vi "Auto_Routine_RightTwoPieceTRAJ.vi"   [LabVIEW 2023]
uses:
  Shoulder/ShoulderGetSetpointEnum.ctl
  Trajectory/TrajectoryGlobals.vi
  <vilib>/Rock Robotics/WPI/ThirdParty/JAS_Junk/TrajLib/Trajectory_Library.lvlib
types:
  T1 = typedef "ShoulderGetSetpointEnum.ctl" = enum16{"ShoulderRest", "ShoulderSpeaker", "ShoulderAmp"}
  T2 = typedef "Trajectory_Library.lvlib/TRAJECTORY.ctl" = cluster{"TotalTImeSecs":dbl, "States":T3[]}
  T3 = typedef "Trajectory_Library.lvlib/TRAJ_STATE.ctl" = cluster{"TimeSeconds":dbl, "Velocity":dbl, "Acceleration":dbl, "POSE":T4, "Curvature":dbl}
  T4 = typedef "Trajectory_Library.lvlib/POSE2D.ctl" = cluster{"TRANSLATION":T5, "ROTATION":T6}
  T5 = typedef "Trajectory_Library.lvlib/TRANSLATION2D.ctl" = cluster{"X":dbl, "Y":dbl}
  T6 = typedef "Trajectory_Library.lvlib/ROTATION2D.ctl" = cluster{"VALUE":dbl, "COS":dbl, "SIN":dbl}
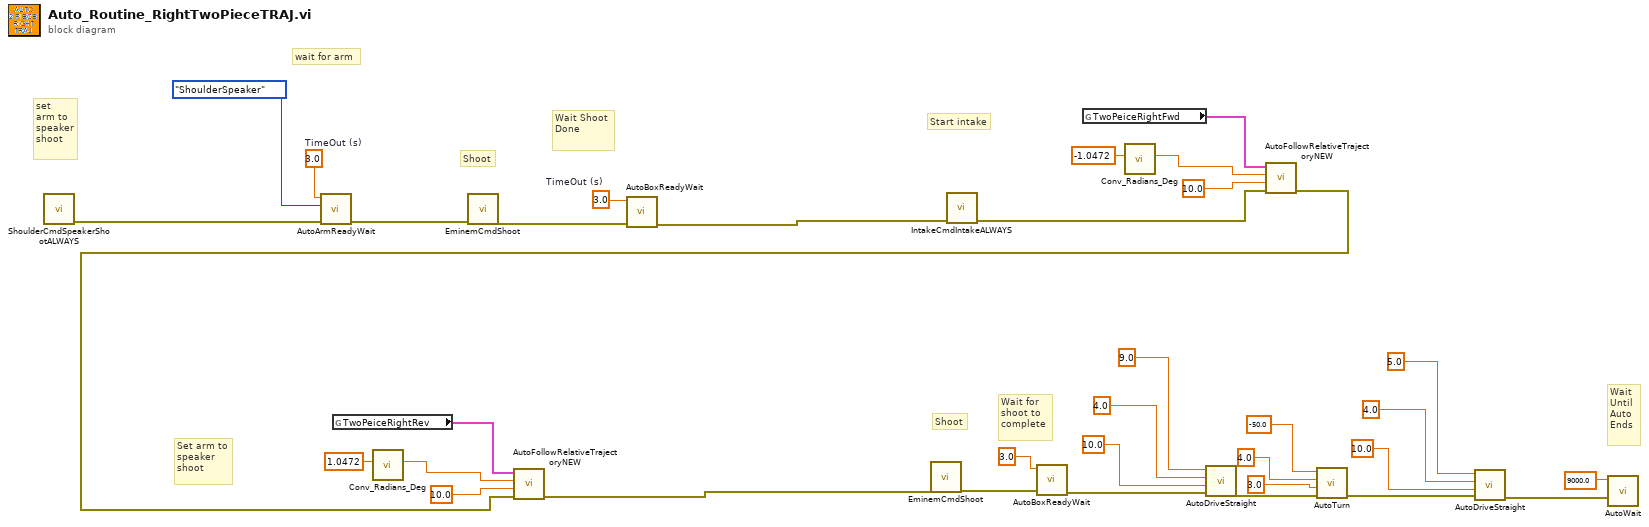
[diagram p0: block diagram]
diagram:
  w34 = 3.0  # TimeOut (s)
  w31 = 3.0  # TimeOut (s)
  # "Wait\nUntil\nAuto \nEnds"
  # "Wait for\nshoot to\ncomplete"
  # "Shoot"
  # "Set arm to\nspeaker \nshoot"
  # "Start intake"
  # "Wait Shoot\nDone"
  # "Shoot"
  # "set \narm to\nspeaker\nshoot"
  # "wait for arm"
  n1 = call "ShoulderCmdSpeakerShootALWAYS.vi"() -> ("error out"=w2:errorcluster)  [unwired: 11 in]
  n2 = call "AutoArmReadyWait.vi"("error in (no error)"=w2, "ArmSetpoints"=ShoulderGetSetpointEnum."ShoulderSpeaker", "TimeOut (s)"=w34) -> ("error out"=w32:errorcluster)  [unwired: 8 in]
  n3 = global read "TrajectoryGlobals.vi" "TwoPeiceRightRev"() -> (w23:T2)
  n4 = call <vilib>:"Conv_Radians_Deg.vi"("Radians"=1.0472) -> ("Degrees"=w21:dbl)  [unwired: 10 in]
  n5 = call "EminemCmdShoot.vi"("error in (no error)"=w32) -> ("error out"=w33:errorcluster)  [unwired: 10 in]
  n6 = call "AutoBoxReadyWait.vi"("error in (no error)"=w33, "TimeOut (s)"=w31) -> ("error out"=w3:errorcluster)  [unwired: 9 in]
  n7 = call "IntakeCmdIntakeALWAYS.vi"("error in (no error)"=w3) -> ("error out"=w5:errorcluster)  [unwired: 10 in]
  n8 = global read "TrajectoryGlobals.vi" "TwoPeiceRightFwd"() -> (w30:T2)
  n9 = call <vilib>:"Conv_Radians_Deg.vi"("Radians"=-1.0472) -> ("Degrees"=w28:dbl)  [unwired: 10 in]
  n10 = call "AutoFollowRelativeTrajectoryNEW.vi"("error in (no error)"=w5, "TimeOut (s)"=10.0, "End Orientation"=w28, "Trajectory"=w30) -> ("error out"=w6:errorcluster)  [unwired: 7 in]
  n11 = call "AutoFollowRelativeTrajectoryNEW.vi"("error in (no error)"=w6, "TimeOut (s)"=10.0, "End Orientation"=w21, "Trajectory"=w23) -> ("error out"=w1:errorcluster)  [unwired: 7 in]
  n12 = call "EminemCmdShoot.vi"("error in (no error)"=w1) -> ("error out"=w25:errorcluster)  [unwired: 10 in]
  n13 = call "AutoBoxReadyWait.vi"("error in (no error)"=w25, "TimeOut (s)"=3.0) -> ("error out"=w19:errorcluster)  [unwired: 9 in]
  n14 = call "AutoDriveStraight.vi"("error in (no error)"=w19, "TimeOut (s)"=10.0, "MaxSpeed (ft/s)"=4.0, "Dist (ft)"=9.0) -> ("error out"=w10:errorcluster)  [unwired: 7 in]
  n15 = call "AutoTurn.vi"("error in (no error)"=w10, "TimeOut (s)"=3.0, "MaxSpeed (ft/s)"=4.0, "degrees"=-50.0) -> ("error out"=w12:errorcluster)  [unwired: 7 in]
  n16 = call "AutoDriveStraight.vi"("error in (no error)"=w12, "TimeOut (s)"=10.0, "MaxSpeed (ft/s)"=4.0, "Dist (ft)"=5.0) -> ("error out"=w11:errorcluster)  [unwired: 7 in]
  n17 = call "AutoWait.vi"("error in (no error)"=w11, "TimeOut (s)"=9000.0) -> ()  [unwired: 9 in, 1 out]
